vi "Process Messages.vi"(8 "error in (no error)":errorcluster, 11 "Deck in":refnum<class "Sample.lvclass">) -> (0 "error out":errorcluster, 3 "Deck out":refnum<class "Sample.lvclass">)   [LabVIEW 2020, in "Sample.lvclass"]
uses:
  Sample.lvclass
  Sample.lvclass/Sample.ctl
  Libraries/Track Info/Track Info.ctl
  Packed Libraries/Messaging.lvlibp/Message Cluster.ctl
  State.ctl
  Packed Libraries/Globals.lvlibp/Constants.vi
  Libraries/Audio File Input/Audio File Input.lvlib
  Packed Libraries/Messaging.lvlibp
  Libraries/User Interface/User Interface.lvlib
  Libraries/Track Info/Track Info.lvlib
  Packed Libraries/Globals.lvlibp
  Packed Libraries/Audio Processing.lvlibp
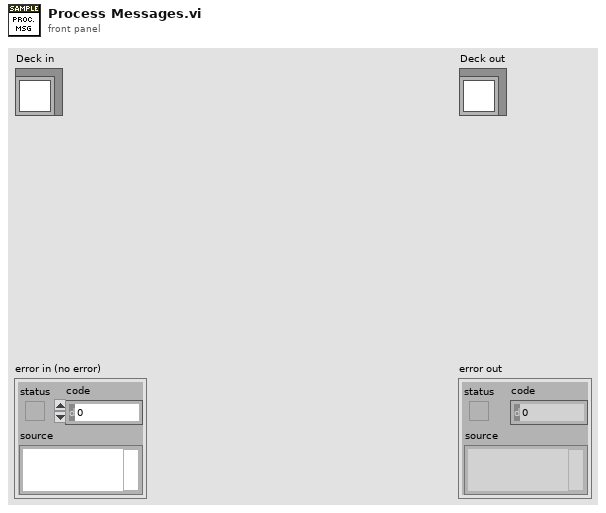
[diagram p1: front panel]
types:
  T1 = typedef "Track Info.lvlib/Track Info.ctl" = cluster{"Path":path, "Length (Samples)":i32, "Channels":i32, "Sample Rate (Hz)":i32, "BPM":dbl, "Cue Points (Samples)":i32[]}
  T2 = typedef "Messaging.lvlibp/Message Cluster.ctl" = cluster{"Event":string, "Source":string, "Target":string, "Data":variant}
  T3 = typedef "Sample.lvclass/State.ctl" = enum16{"No Track", "Loading", "Active", "Scratching", "Brake", "Backspin"}
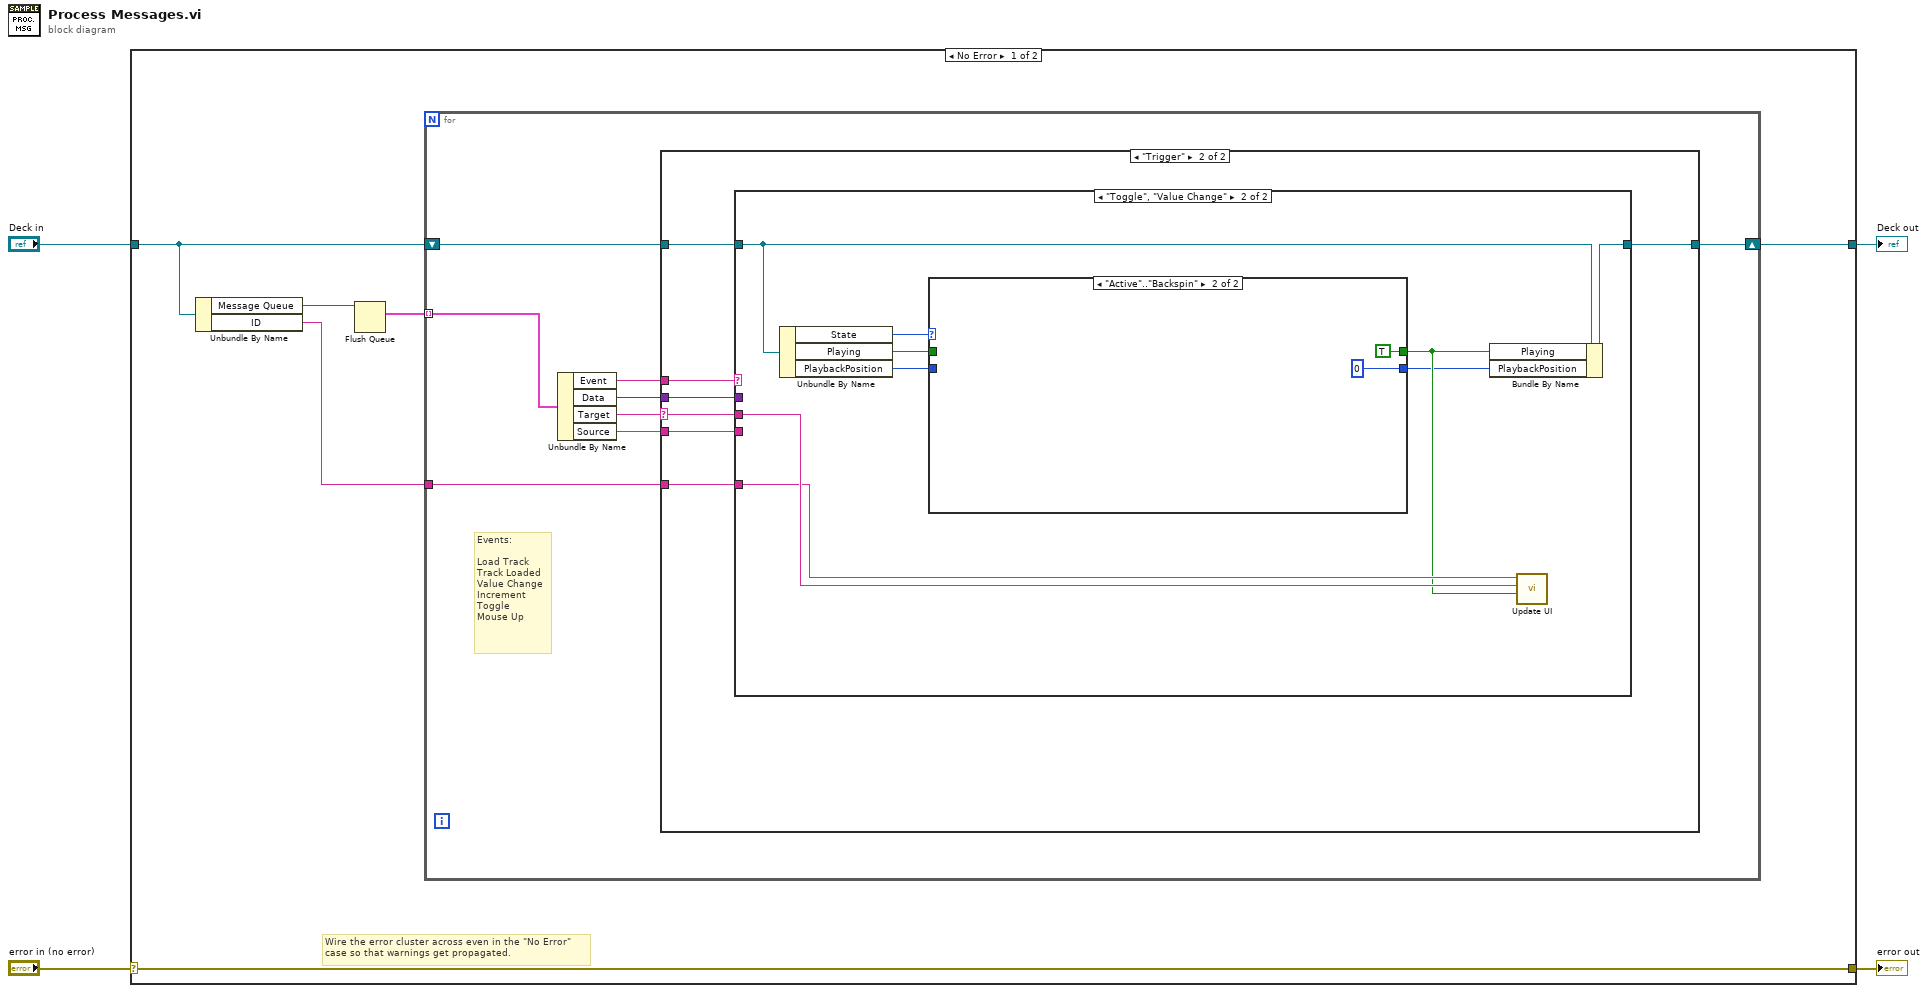
[diagram p0: block diagram]
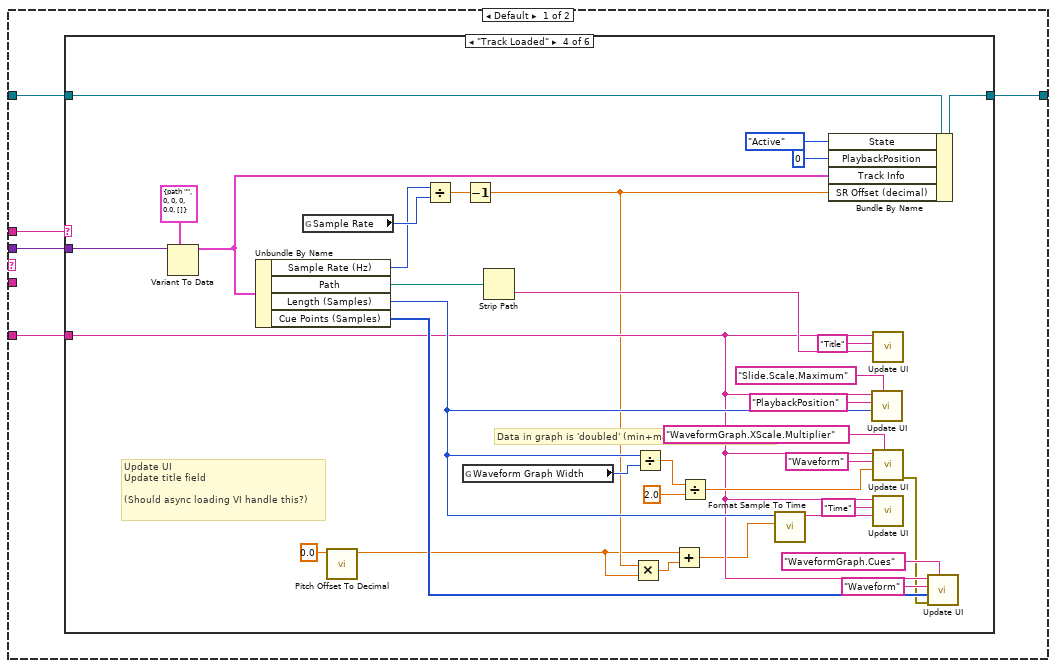
[diagram p2: hidden frame]
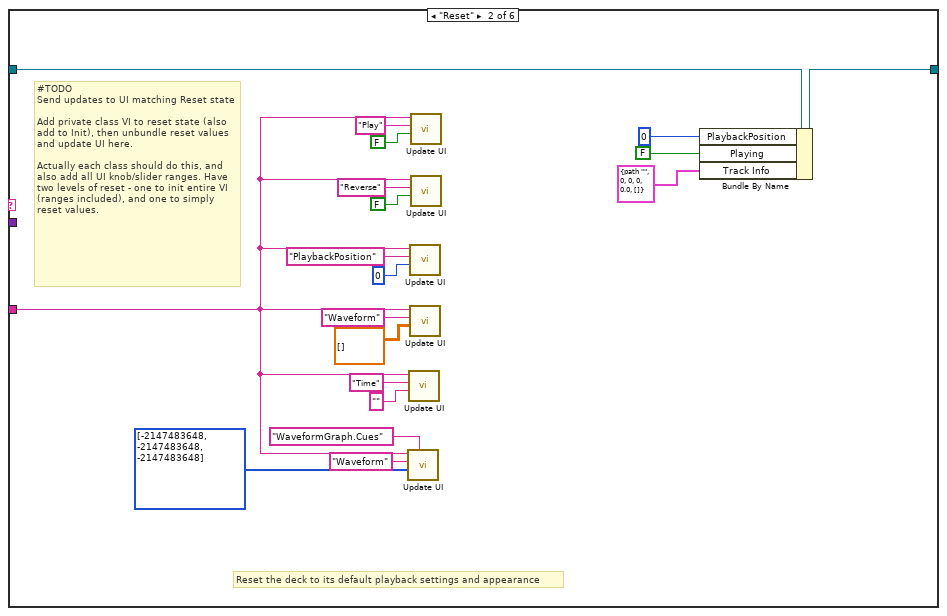
[diagram p4: hidden frame]
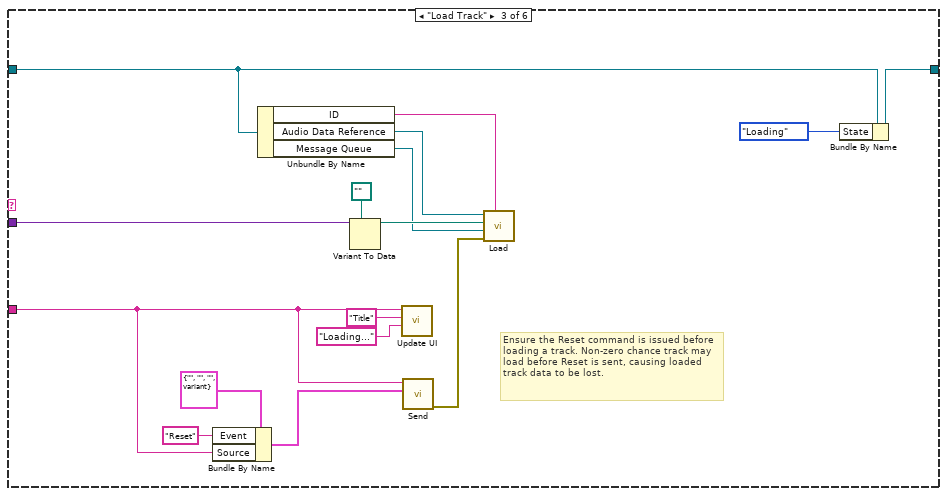
[diagram p5: hidden frame]
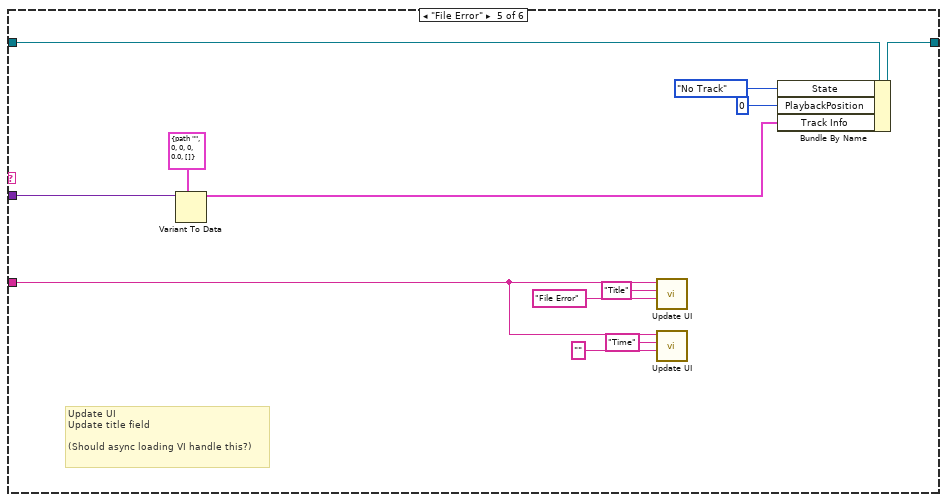
[diagram p6: hidden frame]
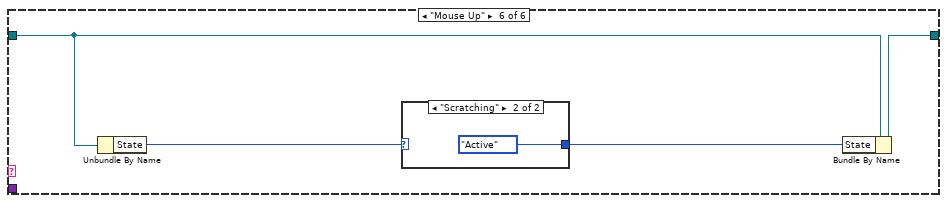
[diagram p7: hidden frame]
diagram:
  n1 = case shown="No Error" "error in (no error)" {
    selector: "error in (no error)" -> [w10 w134]
    tunnel: [w10 w134] -> w3
    tunnel: [w9 w133] -> w1
    tunnel: "Deck in" -> [w8 w133]
    frame No Error {
      # "Wire the error cluster across even in the \"No Error\"\ncase so that warnings get propagated."
      n2 = Unbundle By Name(w8) -> ("Message Queue"=w6:refnum<queue>, "ID"=w7:string)
      n3 = Flush Queue(queue=w6) -> (remaining elements=w5:T2[])  [unwired: 1 in, 2 out]
      n4 = for {
        shift-right: [w16] -> w9
        shift-left: w8 -> [w18]
        tunnel: w7 -> [w14]
        tunnel: w5 -> [w11] mode=indexing
        # "Events:\n\nLoad Track\nTrack Loaded\nValue Change\nIncrement\nToggle\nMouse Up"
        n5 = Unbundle By Name(w11) -> ("Event"=w17:string, "Data"=w15:variant, "Target"=w13:string, "Source"=w12:string)
        n6 = case shown="\"Trigger\"" w13 {
          selector: w13 -> [_ w114]
          tunnel: w18 -> [w23 w118]
          tunnel: w17 -> [w22 w117]
          tunnel: [w21 w116] -> w16
          tunnel: w15 -> [w20 w115]
          tunnel: w14 -> [w19 w113]
          tunnel: w12 -> [_ w112]
          frame Default {
            n7 = case shown="\"Track Loaded\"" w22 {
              tunnel: w23 -> [w24 w36 w52 w65 w103 w106]
              tunnel: [w24 w37 w53 w91 w102 w107] -> w21
              tunnel: w20 -> [_ _ w51 w90 w101 _]
              tunnel: w19 -> [_ w27 w45 w70 w97 _]
              frame Default {
              }
              frame "Reset" {
                # "#TODO\nSend updates to UI matching Reset state\n\nAdd private class VI to reset state (also add to Init), then unbundle reset values and update UI here.\n\nActually each class should do this, and also add all UI knob/slider ranges. Have two levels of reset - one to init entire VI (ranges included), and one to simply reset values."
                # "Reset the deck to its default playback settings and appearance"
                n8 = call "Update UI.vi"("Message (Value Change)"="WaveformGraph.Cues" ("format string"), "Data"=i32[] [-2147483648, -2147483648, -2147483648] ("Cue Points (Samples)"), "Target"="Waveform", "ID"=w27) -> ()  [unwired: 7 in, 1 out]
                n9 = call "Update UI.vi"("Data"="" ("Target"), "Target"="Time", "ID"=w27) -> ()  [unwired: 8 in, 1 out]
                n10 = call "Update UI.vi"("Data"=0, "Target"="PlaybackPosition", "ID"=w27) -> ()  [unwired: 8 in, 1 out]
                n11 = call "Update UI.vi"("Data"=dbl[][] [], "Target"="Waveform", "ID"=w27) -> ()  [unwired: 8 in, 1 out]
                n12 = call "Update UI.vi"("Data"=FALSE ("Playing"), "Target"="Play", "ID"=w27) -> ()  [unwired: 8 in, 1 out]
                n13 = call "Update UI.vi"("Data"=FALSE ("Playing"), "Target"="Reverse", "ID"=w27) -> ()  [unwired: 8 in, 1 out]
                n14 = Bundle By Name(cluster=w36, "PlaybackPosition"=0, "Playing"=FALSE, "Track Info"=T1 {"Path"=path "", "Length (Samples)"=0, "Channels"=0, "Sample Rate (Hz)"=0, "BPM"=0.0, "Cue Points (Samples)"=[]}) -> (w37:refnum<class "Sample.lvclass">)
              }
              frame "Load Track" {
                # "Ensure the Reset command is issued before loading a track. Non-zero chance track may load before Reset is sent, causing loaded track data to be lost."
                n15 = Bundle By Name(cluster=T2 {"Event"="", "Source"="", "Target"="", "Data"=variant} ("Message"), "Event"="Reset", "Source"=w45) -> (w46:T2)
                n16 = Unbundle By Name(w52) -> ("ID"=w59:string, "Audio Data Reference"=w56:refnum<data-value>, "Message Queue"=w55:refnum<queue>)
                n17 = Variant To Data(type=path "", Variant=w51) -> (data=w58:path)  [unwired: 1 in, 1 out]
                n18 = call "Update UI.vi"("Data"="Loading..." ("Target"), "Target"="Title", "ID"=w45) -> ()  [unwired: 8 in, 1 out]
                n19 = call "Send.vi"("Message"=w46, "Queue Name"=w45) -> ("error out"=w44:errorcluster)  [unwired: 9 in]
                n20 = call "Load.vi"("Deck ID"=w59, "error in (no error)"=w44, "Message Queue"=w55, "Path"=w58, "Audio Data Reference"=w56) -> ()  [unwired: 6 in, 1 out]
                n21 = Bundle By Name(cluster=w52, "State"=State."Loading") -> (w53:refnum<class "Sample.lvclass">)
              }
              frame "Track Loaded" {
                # "Data in graph is 'doubled' (min+max for every point)"
                # "Update UI\nUpdate title field\n\n(Should async loading VI handle this?)"
                n22 = Variant To Data(type=T1 {"Path"=path "", "Length (Samples)"=0, "Channels"=0, "Sample Rate (Hz)"=0, "BPM"=0.0, "Cue Points (Samples)"=[]} ("Track Info"), Variant=w90) -> (data=w88:T1)  [unwired: 1 in, 1 out]
                n23 = Unbundle By Name(w88) -> ("Sample Rate (Hz)"=w66:i32, "Path"=w87:path, "Length (Samples)"=w78:i32, "Cue Points (Samples)"=w71:i32[])
                n24 = global read "Constants.vi" "Sample Rate"() -> (w68:i32)
                n25 = call "Pitch Offset To Decimal.vi"("Pitch Offset (%)"=0.0) -> ("Pitch (decimal)"=w62:dbl)  [unwired: 10 in]
                n26 = Divide(x=w66, y=w68) -> (x/y=w67:dbl)
                n27 = global read "Constants.vi" "Waveform Graph Width"() -> (w77:i32)
                n28 = Decrement(x=w67) -> (x-1=w63:dbl)
                n29 = Strip Path(path=w87) -> (name=w86:string)  [unwired: 1 out]
                n30 = Multiply(x=w63, y=w62) -> (x*y=w64:dbl)
                n31 = Divide(x=w78, y=w77) -> (x/y=w76:dbl)
                n32 = Add(x=w62, y=w64) -> (x+y=w61:dbl)
                n33 = Divide(x=w76, y=2.0 ("x")) -> (x/y=w74:dbl)
                n34 = call "Format Sample To Time.vi"("Pitch (decimal) (1)"=w61, "Samples"=w78) -> ("Formatted Time"=w82:string)  [unwired: 9 in]
                n35 = Bundle By Name(cluster=w65, "State"=State."Active", "PlaybackPosition"=0 ("Playback Position (Samples)"), "Track Info"=w88, "SR Offset (decimal)"=w63) -> (w91:refnum<class "Sample.lvclass">)
                n36 = call "Update UI.vi"("Message (Value Change)"="Slide.Scale.Maximum" ("Target"), "Data"=w78, "Target"="PlaybackPosition", "ID"=w70) -> ()  [unwired: 7 in, 1 out]
                n37 = call "Update UI.vi"("Data"=w86, "Target"="Title", "ID"=w70) -> ()  [unwired: 8 in, 1 out]
                n38 = call "Update UI.vi"("Message (Value Change)"="WaveformGraph.XScale.Multiplier" ("Target"), "Data"=w74, "Target"="Waveform", "ID"=w70) -> ("error out"=w69:errorcluster)  [unwired: 7 in]
                n39 = call "Update UI.vi"("Data"=w82, "Target"="Time", "ID"=w70) -> ()  [unwired: 8 in, 1 out]
                n40 = call "Update UI.vi"("Message (Value Change)"="WaveformGraph.Cues" ("format string"), "error in (no error)"=w69, "Data"=w71, "Target"="Waveform", "ID"=w70) -> ()  [unwired: 6 in, 1 out]
              }
              frame "File Error" {
                # "Update UI\nUpdate title field\n\n(Should async loading VI handle this?)"
                n41 = Variant To Data(type=T1 {"Path"=path "", "Length (Samples)"=0, "Channels"=0, "Sample Rate (Hz)"=0, "BPM"=0.0, "Cue Points (Samples)"=[]} ("Track Info"), Variant=w101) -> (data=w99:T1)  [unwired: 1 in, 1 out]
                n42 = call "Update UI.vi"("Data"="File Error" ("Target"), "Target"="Title", "ID"=w97) -> ()  [unwired: 8 in, 1 out]
                n43 = call "Update UI.vi"("Data"="" ("Target"), "Target"="Time", "ID"=w97) -> ()  [unwired: 8 in, 1 out]
                n44 = Bundle By Name(cluster=w103, "State"=State."No Track", "PlaybackPosition"=0 ("Playback Position (Samples)"), "Track Info"=w99) -> (w102:refnum<class "Sample.lvclass">)
              }
              frame "Mouse Up" {
                n45 = Unbundle By Name(w106) -> ("State"=w108:T3)
                n46 = case shown="\"Scratching\"" w108 {
                  selector: w108 -> [w110 _]
                  tunnel: [w110 State."Active" ("State")] -> w109
                  frame Default {
                  }
                  frame "Scratching" {
                  }
                }
                n47 = Bundle By Name(cluster=w106, "State"=w109) -> (w107:refnum<class "Sample.lvclass">)
              }
            }
          }
          frame "Trigger" {
            n48 = case shown="\"Toggle\", \"Value Change\"" w117 {
              tunnel: w118 -> [w119 w127]
              tunnel: [w119 w128] -> w116
              tunnel: w115 -> [_ _]
              tunnel: w114 -> [_ w124]
              tunnel: w113 -> [_ w123]
              tunnel: w112 -> [_ _]
              frame Default {
              }
              frame "Toggle", "Value Change" {
                n49 = Unbundle By Name(w127) -> ("State"=w126:T3, "Playing"=w125:bool, "PlaybackPosition"=w120:i32)
                n50 = case shown="\"Active\"..\"Backspin\"" w126 {
                  tunnel: w125 -> [w130 _]
                  tunnel: [w130 TRUE ("Playing")] -> w122
                  tunnel: [w129 0] -> w121
                  tunnel: w120 -> [w129 _]
                  frame Default {
                  }
                  frame "Active".."Backspin" {
                  }
                }
                n51 = Bundle By Name(cluster=w127, "Playing"=w122, "PlaybackPosition"=w121) -> (w128:refnum<class "Sample.lvclass">)
                n52 = call "Update UI.vi"("Data"=w122, "Target"=w124, "ID"=w123) -> ()  [unwired: 8 in, 1 out]
              }
            }
          }
        }
      }
    }
    frame Error {
    }
  }
  "error out" <- w3
  "Deck out" <- w1
